vi "Load Controller Type from Enum.vi"(8 "error in (no error)":errorcluster, 11 "Controller Type":T1) -> (0 "error out":errorcluster, 3 "controller out":refnum<class "Generic Plugin.lvclass">)   [LabVIEW 2020, in "RxnRover.lvlib" / "Generic Plugin.lvclass"]
uses:
  Generic Plugin.lvclass
  Controller Type.ctl
  Generic Plugin.lvclass/Generic Plugin.ctl
  File IO/File IO.lvlib
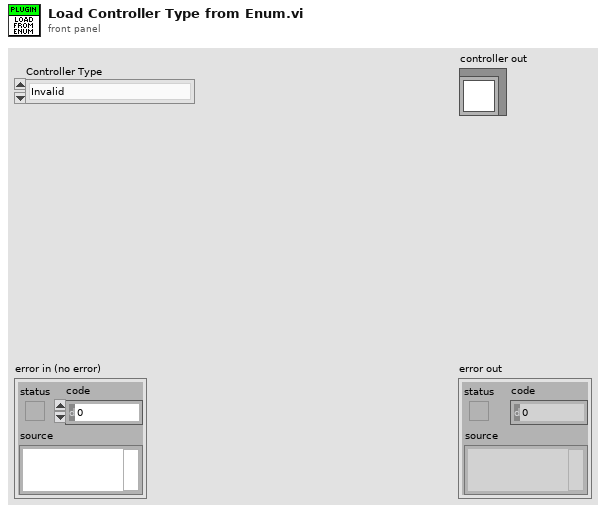
[diagram p1: front panel]
types:
  T1 = typedef "RxnRover.lvlib/Generic Plugin.lvclass/Controller Type.ctl" = enum16{"Invalid", "Temperature Controller", "Pump Controller", "Syringe Pump", "Generic Optimizer", "LC Parser", "Passive Hardware"}
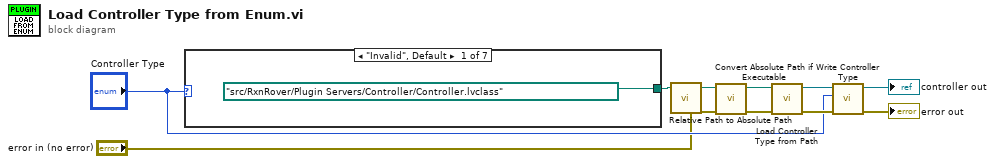
[diagram p0: block diagram]
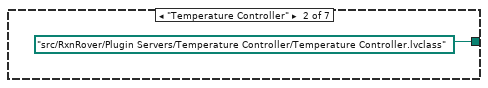
[diagram p2: hidden frame]
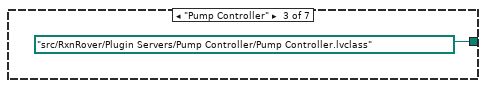
[diagram p3: hidden frame]
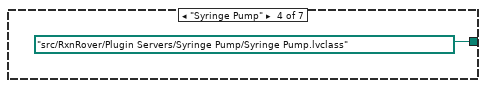
[diagram p4: hidden frame]
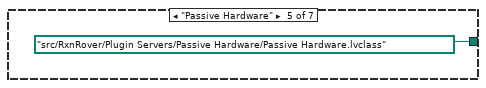
[diagram p5: hidden frame]
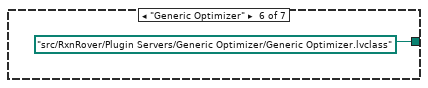
[diagram p6: hidden frame]
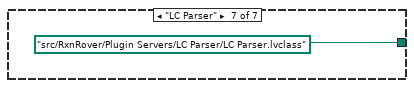
[diagram p7: hidden frame]
diagram:
  n1 = case shown="\"Invalid\", Default" "Controller Type" {
    tunnel: [path "src/RxnRover/Plugin Servers/Controller/Controller.lvclass" path "src/RxnRover/Plugin Servers/Temperature Controller/Temperature Controller.lvclass" path "src/RxnRover/Plugin Servers/Pump Controller/Pump Controller.lvclass" path "src/RxnRover/Plugin Servers/Syringe Pump/Syringe Pump.lvclass" path "src/RxnRover/Plugin Servers/Passive Hardware/Passive Hardware.lvclass" path "src/RxnRover/Plugin Servers/Generic Optimizer/Generic Optimizer.lvclass" path "src/RxnRover/Plugin Servers/LC Parser/LC Parser.lvclass"] -> w10
    frame "Invalid", Default {
    }
    frame "Temperature Controller" {
    }
    frame "Pump Controller" {
    }
    frame "Syringe Pump" {
    }
    frame "Passive Hardware" {
    }
    frame "Generic Optimizer" {
    }
    frame "LC Parser" {
    }
  }
  n2 = call "Relative Path to Absolute Path.vi"("Relative Path"=w10) -> ("Absolute Path"=w4:path)  [unwired: 4 in]
  n3 = call "Convert Absolute Path if Executable.vi"("error in (no error)"="error in (no error)", "Absolute Path"=w4) -> ("error out"=w1:errorcluster, "Result Path"=w3:path)  [unwired: 7 in, 1 out]
  n4 = call "Load Controller Type from Path.vi"("error in (no error)"=w1, "Class Path"=w3) -> ("error out"=w7:errorcluster, "Controller out"=w9:refnum<class "Generic Plugin.lvclass">)
  n5 = call "Write Controller Type.vi"("error in (no error)"=w7, "Controller Type"="Controller Type", "Generic Controller in"=w9) -> ("error out"=→"error out":errorcluster, "Generic Controller out"=→"controller out":refnum<class "Generic Plugin.lvclass">)  [unwired: 7 in]
